vi "TEST_bench_hysteresis_fxp_16_5.vi"(7 "N_hyst":i32) -> ()   [LabVIEW 2017]
uses:
  <vilib>/Platform/TimedLoop/XDataNode/timing_clust.ctl
  <vilib>/Platform/TimedLoop/XDataNode/nitl_modes.ctl
  <vilib>/Platform/TimedLoop/XDataNode/wakeup.ctl
  <vilib>/rvi/Emulation/niFpgaSctlEmulationGetInTimedLoop.vi
  <vilib>/rvi/Emulation/niFpgaEmulationReportErrorSimple.vi
  <vilib>/rvi/Emulation/niFpgaGetClockAttributes.vi
  <vilib>/rvi/Emulation/niFpgaCriticalErrorInLSC.vi
  <vilib>/rvi/Memory/Memory_Emulation/nirvimemoryFastEmulation.vi
  <vilib>/rvi/Memory/Memory_Emulation/nirvimemoryEmulation.vi
  <vilib>/rvi/Emulation/niFpgaEmulationIsFPGAContextNoSignature.vi
  <vilib>/rvi/DataTransferAndStorage/Container/Common/niFpgaContainerGetUniqueNameForEmu.vi
  <vilib>/rvi/Emulation/niFpgaProcessEmulError.vi
  <vilib>/rvi/errors/nirviReportUnexpectedCaseInternalError (U32).vi
  <vilib>/Platform/TimedLoop/XDataNode/XDataNode.xnode
  <vilib>/rvi/DataTransferAndStorage/Container/XNode/niFpgaContainer.xnode
  <vilib>/Platform/TimedLoop/XDataNode/XDNodeRunTimeDep.lvlib
panel:
  out "H_of_ik (expected)":sgl[](array[numeric])
  out "H_of_uk":fxp<+/-,32,10>[](array[numeric])
  in  "uk":sgl[](array[numeric]) format="%#_13g"
  in  "numIter":i32
  out "y_vec_out (expected)":sgl[](array[numeric])
  out "y_out_mem":fxp<+/-,16,5>[](array[numeric])
  in  "y_vec_in":fxp<+/-,16,5>[](array[numeric])=[0.0, 0.0, 0.0, 0.0, 0.0, 0.0, 0.0]
  in  "r_s":fxp<+/-,16,5>[](array[numeric])=[0.0, 0.82861328125, 1.8125, 2.8671875, 4.03173828125, 5.2001953125, 7.20166015625]
  in  "w_s":fxp<+/-,16,5>[](array[numeric])=[0.0, 0.0, 0.0, 0.0, 0.0, 0.0, 0.0]
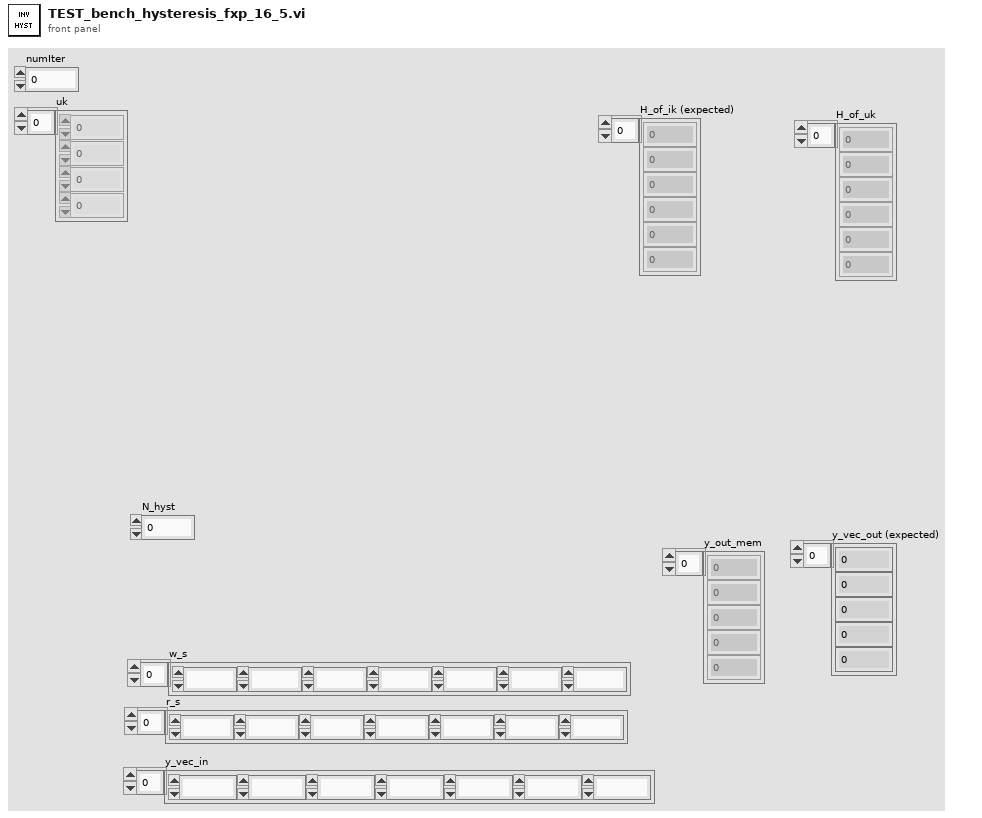
[diagram p1: front panel]
types:
  T1 = typedef "XDNodeRunTimeDep.lvlib/timing_clust.ctl" = cluster{"Expected End [f-1]":u64, "Actual End [f-1]":u64, "Finished Late? [f-1]":bool, "Expected End [i-1]":u64, "Actual End [i-1]":u64, "Finished Late? [i-1]":bool, "Expected Start [i]":u64, "Actual Start [i]":u64, "Expected Start [f]":u64, "Actual Start [f]":u64, "Source Name":string, "Structure Name":string, "Period":i64, "Deadline":i64, "Offset":i64, "Start":i64, "Priority":i32, "Timeout":i32, "Mode":T2, "Wakeup Reason":T3, "Error":errorcluster, "Source Type":string, "Secondary Source Type":string, "Global End Time":u64, "Global Start Time":u64, "Frame Duration":u64, "Iteration Duration":u64, "Assigned CPU":i32, "I/O Scan Engine Mode":u32}
  T2 = typedef "XDNodeRunTimeDep.lvlib/nitl_modes.ctl" = enum32{"No Change", "Process missed periods, maintain original phase", "Discard missed periods, maintain original phase", "Process missed periods, ignore original phase", "Discard missed periods, ignore original phase"}
  T3 = typedef "XDNodeRunTimeDep.lvlib/wakeup.ctl" = enum32{"Normal", "Aborted", "Asynchronous wakeup", "Timing source error", "Timed loop error", "Timeout"}
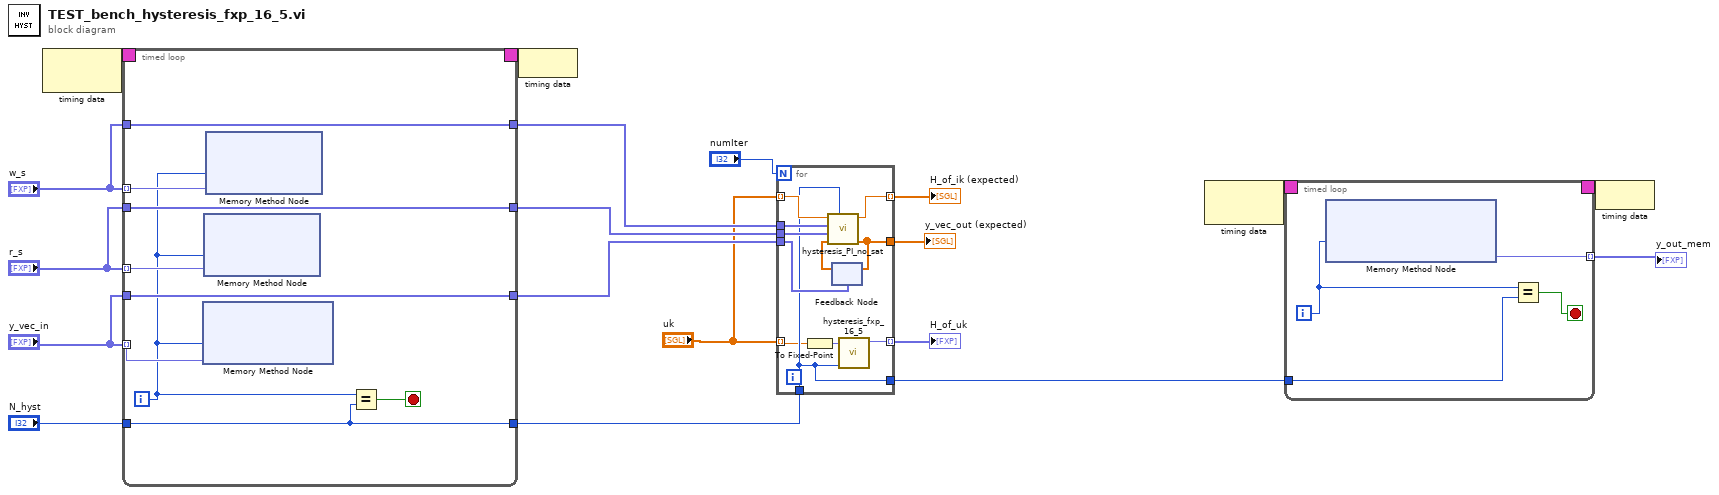
[diagram p0: block diagram]
diagram:
  n1 = node-c288() -> (w16:T1)  [unwired: 1 in]
  n2 = timed-loop {
    timing: w16 -> [_]
    timing-out: [_] -> w15
    tunnel: "w_s" -> [w27] mode=indexing
    tunnel: "r_s" -> [w25] mode=indexing
    tunnel: "y_vec_in" -> [w26] mode=indexing
    tunnel: [w24] -> w12
    tunnel: "w_s" -> [w24]
    tunnel: [w23] -> w11
    tunnel: "r_s" -> [w23]
    tunnel: [w22] -> w10
    tunnel: "y_vec_in" -> [w22]
    tunnel: "N_hyst" -> [w20]
    tunnel: [w20] -> w5
    i -> [w21]
    stop <- w28 stop-if-true
    n3 = xnode ("Memory Method Node")("Address"=w21, "Data"=w26) -> ()  [unwired: 1 in, 1 out]
    n4 = xnode ("Memory Method Node")("Address"=w21, "Data"=w25) -> ()  [unwired: 1 in, 1 out]
    n5 = xnode ("Memory Method Node")("Address"=w21, "Data"=w27) -> ()  [unwired: 1 in, 1 out]
    n6 = Equal?(x=w21, y=w20) -> (x = y?=w28:bool)
  }
  n7 = node-c288(w15) -> ()
  n8 = for {
    N: "numIter" -> [_]
    tunnel: "uk" -> [w31] mode=indexing
    tunnel: [w41] -> w2 mode=indexing
    tunnel: w12 -> [w39]
    tunnel: w11 -> [w38]
    tunnel: w10 -> [w34]
    tunnel: [w35] -> w9
    tunnel: w5 -> [w33]
    tunnel: "uk" -> [w40] mode=indexing
    tunnel: [w37] -> w1 mode=indexing
    tunnel: [w33] -> w4
    n9 = To Fixed-Point(number=w31) -> (fixed-point=w32:fxp<+/-,16,5>)  [unwired: 1 in]
    n10 = feedback #1(w34) -> (w36:sgl[])
    n11 = call "hysteresis_PI_no_sat.vi"("N_hyst"=w33, "y_vec_in"=w36, "r_s"=w38, "w_s"=w39, "uk"=w40) -> ("y_vec_out"=w35:sgl[], "H_of_ik"=w37:sgl)  [unwired: 5 in]
    n12 = feedback-in #1(w35) -> ()
    n13 = call "hysteresis_fxp_16_5.vi"("N_hyst"=w33, "uk_in"=w32) -> ("Hinv(uk)"=w41:fxp<+/-,32,10>)  [unwired: 9 in]
  }
  "y_vec_out (expected)" <- w9
  "H_of_uk" <- w2
  "H_of_ik (expected)" <- w1
  n14 = node-c288() -> (w19:T1)  [unwired: 1 in]
  n15 = timed-loop {
    timing: w19 -> [_]
    timing-out: [_] -> w18
    tunnel: [w45] -> w17 mode=indexing
    tunnel: w4 -> [w42]
    i -> [w43]
    stop <- w44 stop-if-true
    n16 = xnode ("Memory Method Node")("Address"=w43) -> ("Data"=w45:fxp<+/-,16,5>)  [unwired: 1 in, 1 out]
    n17 = Equal?(x=w43, y=w42) -> (x = y?=w44:bool)
  }
  "y_out_mem" <- w17
  n18 = node-c288(w18) -> ()
